vi "Configure Clock Recovery (Explicit).vi"(6 "Edges (0: Rising)":u16(ring) items=["Rising", "Falling", "Either"], 7 "Enable Clock Recovery (T: Enable)":bool=TRUE, 8 "error in (no error)":errorcluster, 9 "Multiplier (1)":i32=1, 10 "Source (1: Channel 1)":u16(ring)=1 items=["Channel 1"=1, "Channel 2"=2, "Channel 3"=3, "Channel 4"=4], 11 "VISA resource name":refnum<visa-resource-name>) -> (0 "error out":errorcluster, 3 "VISA resource name out":refnum<visa-resource-name>)   [LabVIEW 2015, in "Agilent 2000 3000 X-Series.lvlib"]
doc: "Configures clock recovery, the clock is recovered from a second signal in your device under test, with a multiplier from 1 to 1000 applied.\n\n<b>Note:</b>\nThis VI is specific to the 6000-X Series oscilloscopes. These features are not available on other models. Use <b>Configure Math Function Characteristics</b> and <b>Configure Math Function Source</b> before running this vi to set <b>Clock Recovery</b> as the math function and select the desired source."
uses:
  Agilent 2000 3000 X-Series.lvlib
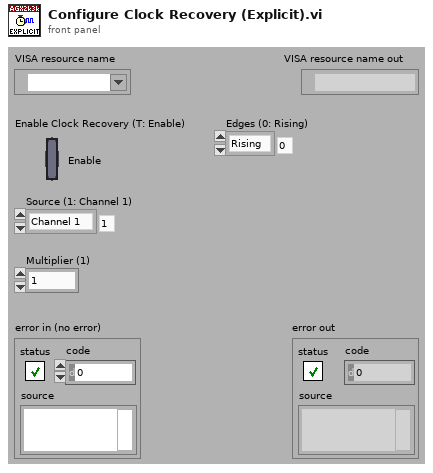
[diagram p1: front panel]
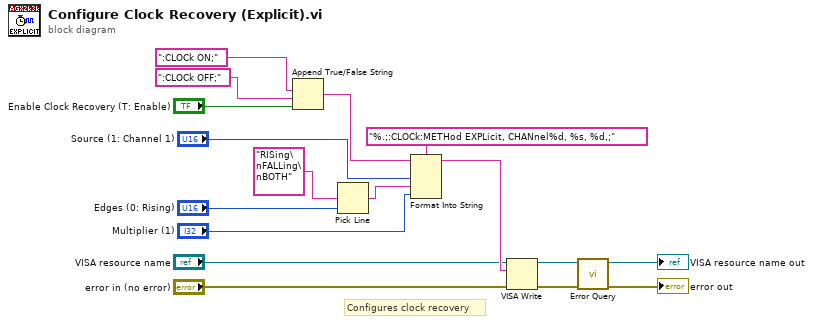
[diagram p0: block diagram]
diagram:
  # "Configures clock recovery"
  n1 = Append True/False String(1:"Enable Clock Recovery (T: Enable)", 2:":CLOCk OFF;", 3:":CLOCk ON;") -> (0:w14:string)  [unwired: 1 in]
  n2 = Pick Line(multi-line string="RISing\nFALLing\nBOTH", line index="Edges (0: Rising)") -> (output string=w6:string)  [unwired: 1 in]
  n3 = Format Into String(format string="%.;:CLOCk:METHod EXPLicit, CHANnel%d, %s, %d,;", initial string=w14, "Source (1: Channel 1)", w6, "Multiplier (1)") -> (resulting string=w13:string)  [unwired: 1 in, 1 out]
  n4 = VISA Write(VISA resource name="VISA resource name", write buffer=w13, error in (no error)="error in (no error)") -> (VISA resource name out=w4:refnum<visa-resource-name>, error out=w3:errorcluster)  [unwired: 1 out]
  n5 = call "Error Query.vi"("error in (no error)"=w3, "VISA resource name"=w4) -> ("error out"=→"error out":errorcluster, "VISA resource name out"=→"VISA resource name out":refnum<visa-resource-name>)  [unwired: 6 in, 2 out]
